vi "setConfiguration.vi"(8 "error in (no error)":errorcluster, 10 "Configuration":variant, 11 "Instrument in":refnum<class "Instrument.lvclass">) -> (0 "error out":errorcluster, 3 "Instrument out":refnum<class "Instrument.lvclass">)   [LabVIEW 2019, in "Instrument.lvclass"]
doc: "Set \"setConfiguration\" to remote Instrument process."
uses:
  Instrument.lvclass
  Typedefs/Instrument.ProtectedCommands--Enum.ctl
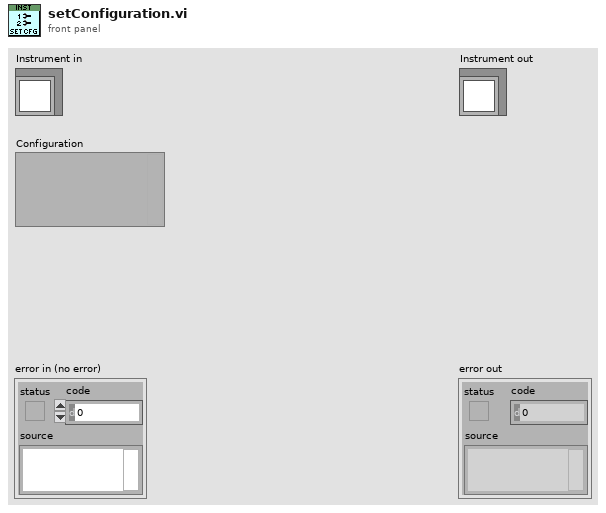
[diagram p1: front panel]
types:
  T1 = typedef "Instrument.lvclass/Instrument.ProtectedCommands--Enum.ctl" = enum16{"setConfiguration", "setLogData", "setIDN", "setAll", "setAllData"}
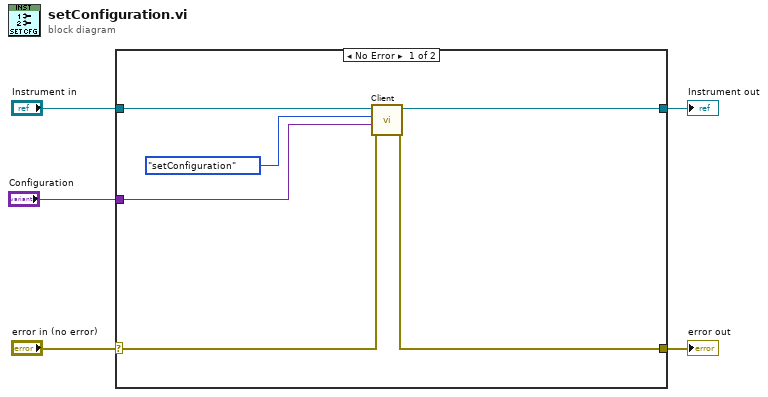
[diagram p0: block diagram]
diagram:
  n1 = case shown="No Error" "error in (no error)" {
    selector: "error in (no error)" -> [w9 w13]
    tunnel: [w8 w13] -> w4
    tunnel: [w7 w12] -> w2
    tunnel: "Instrument in" -> [w11 w12]
    tunnel: "Configuration" -> [w10 _]
    frame No Error {
      n2 = call-dynamic "Client.vi"("error in (no error)"=w9, "Data in"=w10, "Command in"=Instrument.ProtectedCommands--Enum."setConfiguration" ("PrivateCommands"), "Instrument in"=w11) -> ("error out"=w8:errorcluster, "Instrument out"=w7:refnum<class "Instrument.lvclass">)  [unwired: 4 in, 2 out]
    }
    frame Error {
    }
  }
  "error out" <- w4
  "Instrument out" <- w2
